vi "SensorMode1.vi"(10 "Numeric":i16, 11 "Numeric 2":i16) -> (1 "Sensor OK 4":bool, 2 "Sensor OK 5":bool, 3 "Sensor OK 6":bool, 4 "Sensor OK 3":bool)   [LabVIEW 2017]
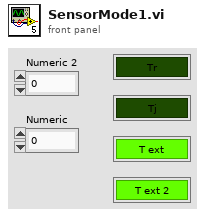
[diagram p1: front panel]
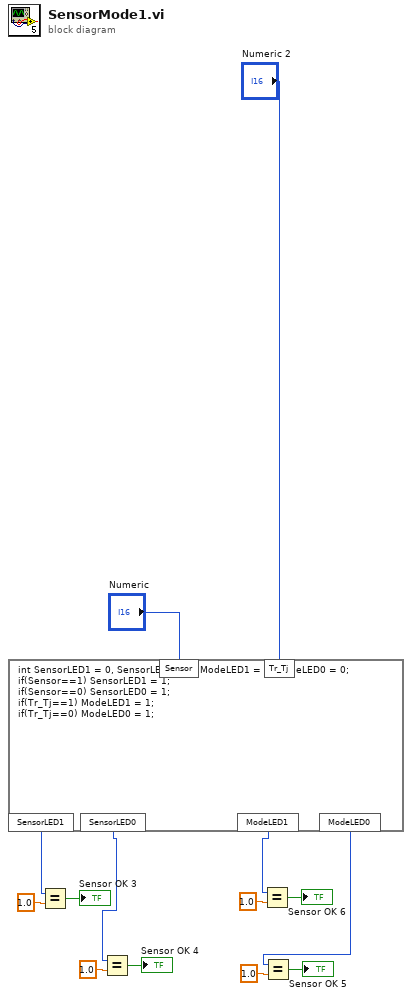
[diagram p0: block diagram]
diagram:
  n1 = formula code="int SensorLED1 = 0, SensorLED0 = 0, ModeLED1 = 0, ModeLED0 = 0;\nif(Sensor==1) SensorLED1 = 1;\nif(Sensor==0) SensorLED0 = 1;\nif(Tr_Tj==1) ModeLED1 = 1;\nif(Tr_Tj==0) ModeLED0 = 1;"("Tr_Tj"="Numeric 2", "Sensor"="Numeric") -> ("SensorLED1"=w3:i32, "SensorLED0"=w5:i32, "ModeLED1"=w14:i32, "ModeLED0"=w10:i32)
  n2 = Equal?(x=w3, y=1.0) -> (x = y?=→"Sensor OK 3":bool)
  n3 = Equal?(x=w5, y=1.0) -> (x = y?=→"Sensor OK 4":bool)
  n4 = Equal?(x=w14, y=1.0) -> (x = y?=→"Sensor OK 6":bool)
  n5 = Equal?(x=w10, y=1.0) -> (x = y?=→"Sensor OK 5":bool)
